vi "cRIO UDP test.vi"() -> ()   [LabVIEW 2009]
uses:
  UDP Lib/UDP Network Location.ctl
panel:
  in  "GO":bool
  in  "Destination Location":T1
  in  "Send Data":string
  in  "stop":bool
  out "Timeout":bool
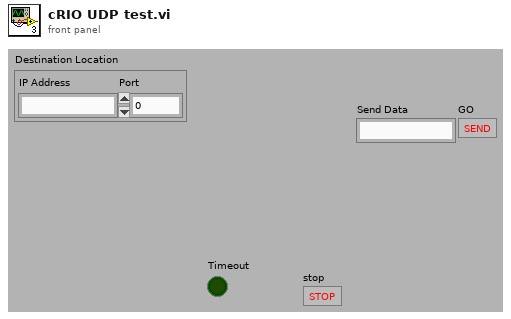
[diagram p1: front panel]
types:
  T1 = typedef "UDP Network Location.ctl" = cluster{"IP Address":string, "Port":u16}
  T2 = typedef "UDP Base.ctl" = cluster{"UDP Session":refnum<k16>, "UDP Socket Params":T3}
  T3 = typedef "UDP Socket Params.ctl" = cluster{"Local Port":u16, "Read Timeout":i32, "Write Timeout":i32}
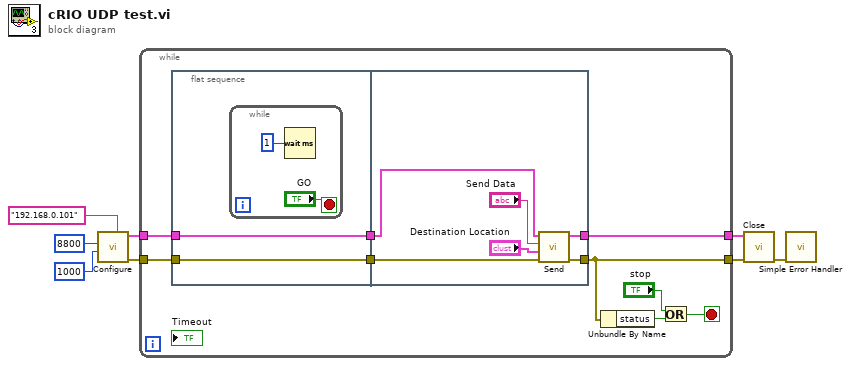
[diagram p0: block diagram]
diagram:
  n1 = call "Configure.vi"("net address"="192.168.0.101", "Read Timeout"=1000, "Local Port"=u16 8800) -> ("error out"=w7:errorcluster, "UDP Base out"=w8:T2)  [unwired: 7 in]
  n2 = while {
    tunnel: w8 -> [w14]
    tunnel: w7 -> [w13]
    tunnel: [w12] -> w3
    tunnel: [w11] -> w4
    stop <- w16 stop-if-true
    n3 = flat-sequence {
      tunnel: w13 -> [w18]
      tunnel: w14 -> [w19]
      tunnel: [w19] -> w10
      tunnel: [w18] -> w9
      tunnel: [w25] -> w12
      tunnel: [w24] -> w11
      tunnel: w10 -> [w27]
      tunnel: w9 -> [w26]
      frame #0 {
        n4 = while {
          stop <- "GO" stop-if-true
          n5 = Wait (ms)(milliseconds to wait=u32 1) -> ()  [unwired: 1 out]
        }
      }
      frame #1 {
        n6 = call "Send.vi"("error in (no error)"=w26, "Destination Location"="Destination Location", "Send Data"="Send Data", "UDP Base in"=w27) -> ("error out"=w25:errorcluster, "UDP Base out"=w24:T2)  [unwired: 5 in, 1 out]
      }
    }
    n7 = Unbundle By Name(w12) -> ("status"=w15:bool)
    n8 = Or(x="stop", y=w15) -> (x .or. y?=w16:bool)
  }
  n9 = call "Close.vi"("error in (no error)"=w3, "Cluster of class private data"=w4) -> ("error out"=w2:errorcluster)  [unwired: 9 in]
  n10 = call <vilib>:"Simple Error Handler.vi"("error in (no error)"=w2) -> ()  [unwired: 4 in, 5 out]
